vi "Fire User Event - Stop.vi"(8 "Error In":errorcluster) -> (0 "Error Out":errorcluster)   [LabVIEW 2017]
doc: "Send the Stop event to stop the Event Handling Loop."
uses:
  Global Variables/gl_User Events.vi
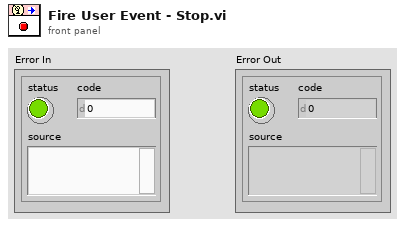
[diagram p1: front panel]
types:
  T1 = cluster{"User Event - Stop":refnum<user-event>, "User Event - Next State":refnum<user-event>}
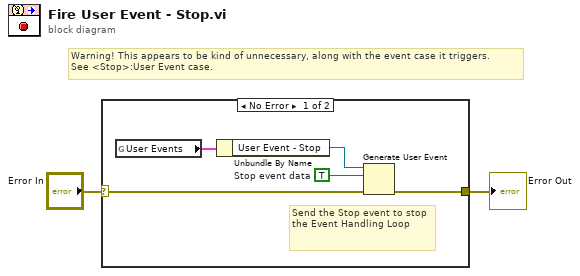
[diagram p0: block diagram]
diagram:
  # "Warning! This appears to be kind of unnecessary, along with the event case it triggers.\nSee <Stop>:User Event case."
  n1 = case shown="No Error" "Error In" {
    selector: "Error In" -> [w5 w8]
    tunnel: [w6 w8] -> w1
    frame No Error {
      w7 = TRUE  # Stop event data
      # "Send the Stop event to stop the Event Handling Loop"
      n2 = global read "gl_User Events.vi" "User Events"() -> (w4:T1)
      n3 = Unbundle By Name(w4) -> ("User Event - Stop"=w3:refnum<user-event>)
      n4 = Generate User Event(user event=w3, event data cluster=w7, error in=w5) -> (error out=w6:errorcluster)  [unwired: 1 in, 1 out]
    }
    frame Error {
    }
  }
  "Error Out" <- w1
